vi "GAIN BASIC.vi"(0 "SR850 GPIB In":refnum<visa-resource-name>, 1 "Max. Hassasiyet":dbl=15.0, 2 "Auto Gain (False)":bool, 9 "Min. Hassasiyet":u16(ring) items=["100 nV", "200 nV", "500 nV", "1 uV", "2 uV", "5 uV", "10 uV", "20 uV", "50 uV", "100 uV", "200 uV", "500 uV", "1 mV"], 11 "error in":errorcluster) -> (4 "SR850 GPIB Out":refnum<visa-resource-name>, 15 "error out":errorcluster)   [LabVIEW 2014]
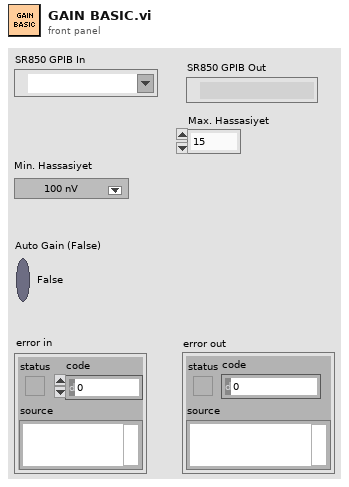
[diagram p1: front panel]
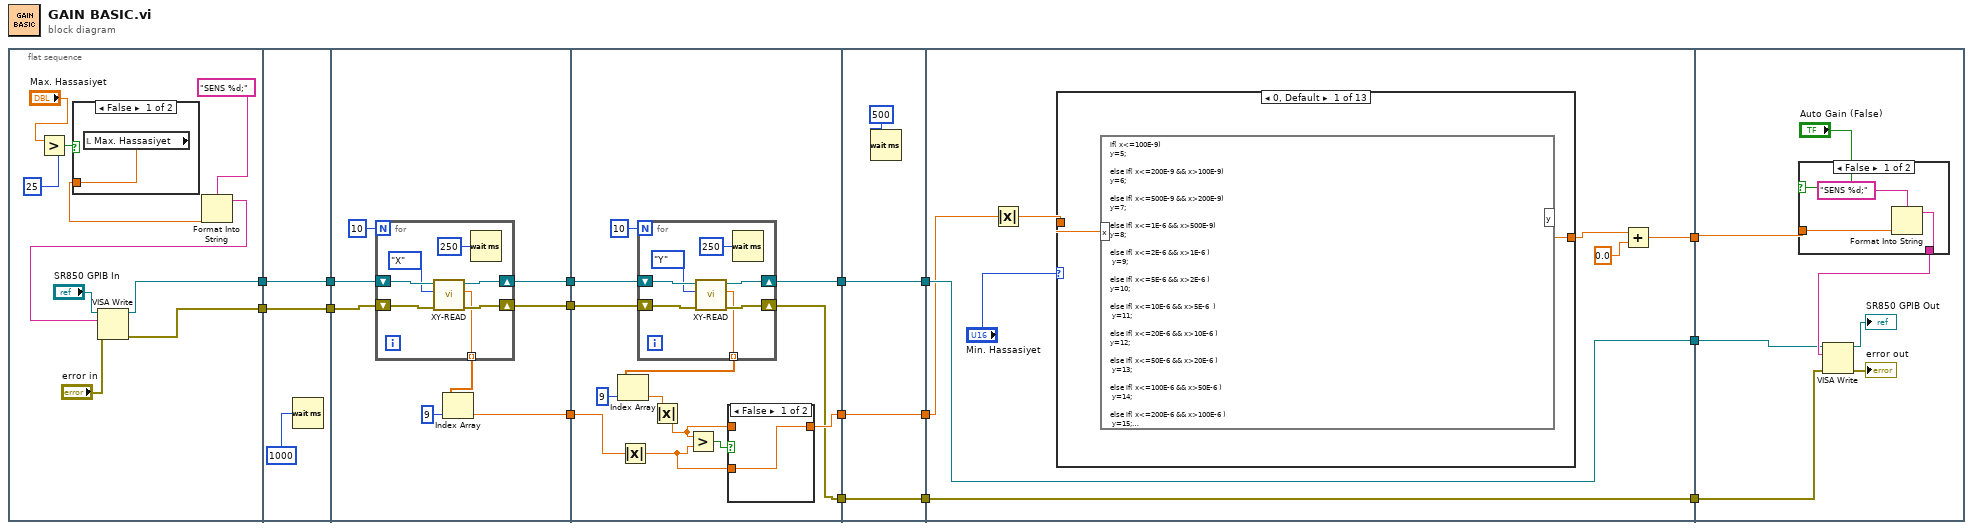
[diagram p0: block diagram]
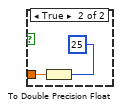
[diagram p2: hidden frame]
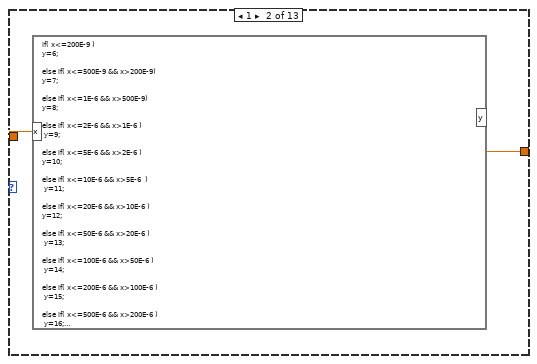
[diagram p4: hidden frame]
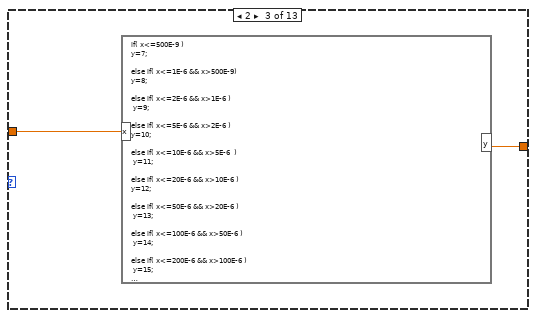
[diagram p5: hidden frame]
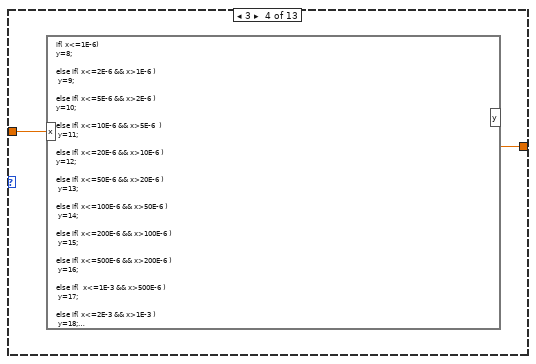
[diagram p6: hidden frame]
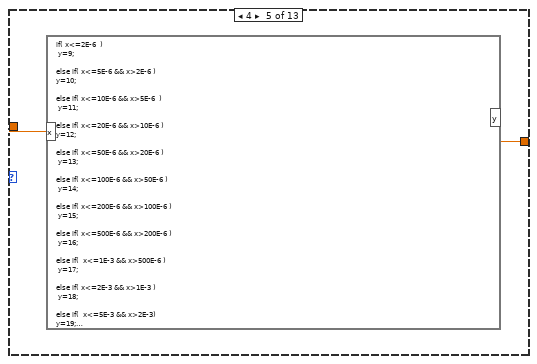
[diagram p7: hidden frame]
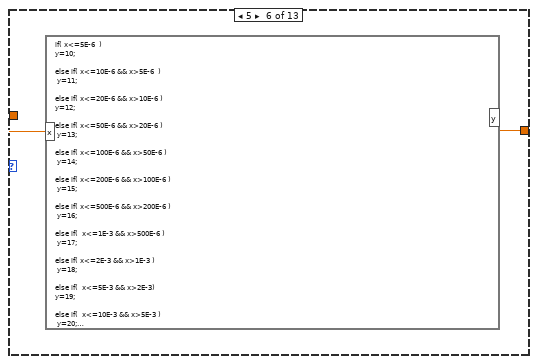
[diagram p8: hidden frame]
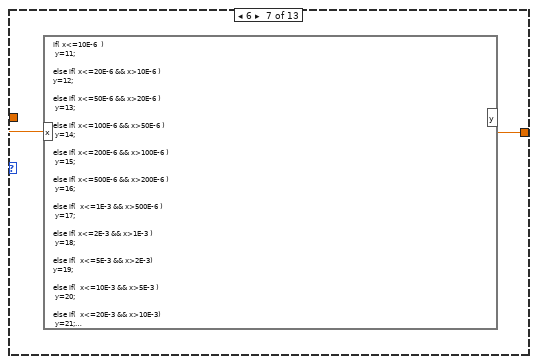
[diagram p9: hidden frame]
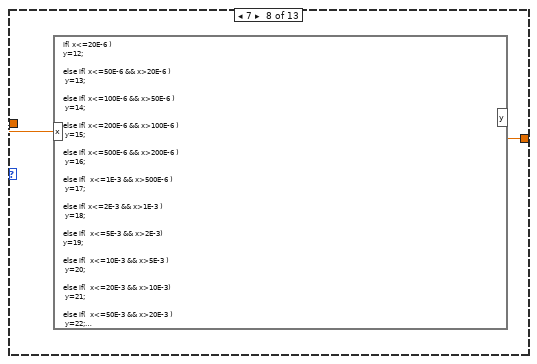
[diagram p10: hidden frame]
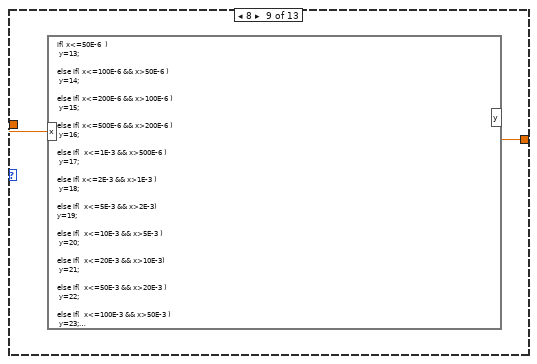
[diagram p11: hidden frame]
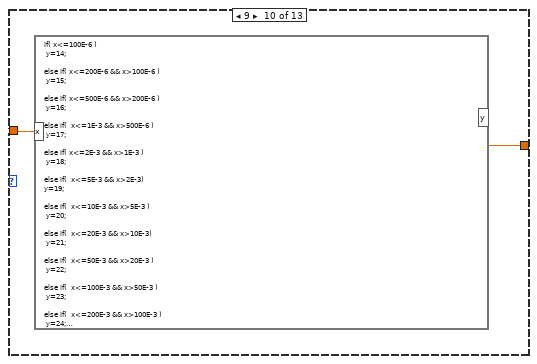
[diagram p12: hidden frame]
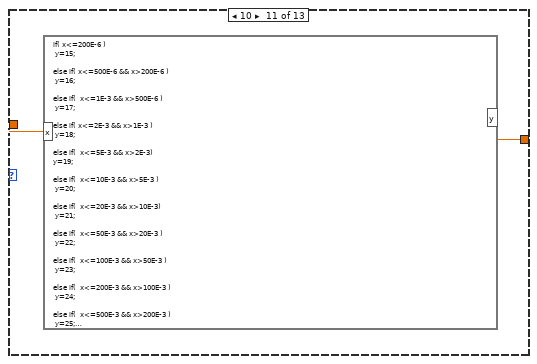
[diagram p13: hidden frame]
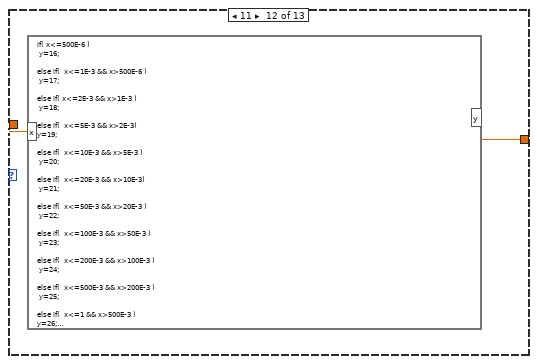
[diagram p14: hidden frame]
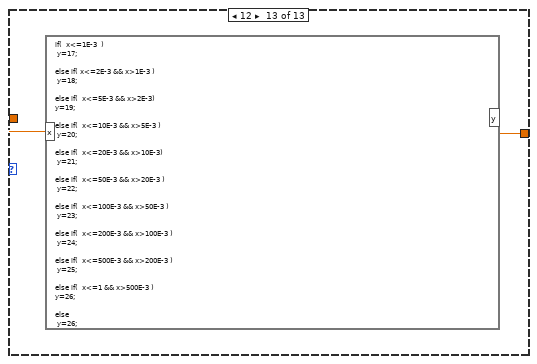
[diagram p15: hidden frame]
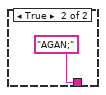
[diagram p16: hidden frame]
diagram:
  n1 = flat-sequence {
    tunnel: [w24] -> w13
    tunnel: [w21] -> w11
    tunnel: w13 -> [w32]
    tunnel: [w32] -> w12
    tunnel: w11 -> [w31]
    tunnel: [w31] -> w10
    tunnel: w12 -> [w40]
    tunnel: w10 -> [w39]
    tunnel: [w38] -> w6
    tunnel: [w34] -> w3
    tunnel: [w33] -> w1
    tunnel: w6 -> [w56]
    tunnel: [w57] -> w5
    tunnel: [w48] -> w4
    tunnel: w3 -> [w52]
    tunnel: [w51] -> w2
    tunnel: w1 -> [w55]
    tunnel: w5 -> [w73]
    tunnel: [w73] -> w9
    tunnel: w4 -> [w72]
    tunnel: [w72] -> w8
    tunnel: w2 -> [w71]
    tunnel: [w71] -> w7
    tunnel: [w80] -> w16
    tunnel: w9 -> [w80]
    tunnel: [w79] -> w15
    tunnel: w8 -> [w79]
    tunnel: w7 -> [w77]
    tunnel: [w74] -> w14
    tunnel: w16 -> [w109]
    tunnel: w15 -> [w108]
    tunnel: w14 -> [w110]
    frame #0 {
      n2 = Greater?(x="Max. Hassasiyet", y=25) -> (0:w18:bool)
      n3 = case shown="False" w18 {
        tunnel: [w27 w28] -> w17
        frame False {
          n4 = local read "Max. Hassasiyet"() -> (w27:dbl)
        }
        frame True {
          n5 = To Double Precision Float(number=25) -> (double precision float=w28:dbl)
        }
      }
      n6 = Format Into String(format string="SENS %d;", w17) -> (resulting string=w22:string)  [unwired: 2 in, 1 out]
      n7 = VISA Write(VISA resource name="SR850 GPIB In", write buffer=w22, error in (no error)="error in") -> (VISA resource name out=w24:refnum<visa-resource-name>, error out=w21:errorcluster)  [unwired: 1 out]
    }
    frame #1 {
      n8 = Wait (ms)(milliseconds to wait=u32 1000) -> ()  [unwired: 1 out]
    }
    frame #2 {
      n9 = for {
        N: 10 -> [_]
        shift-right: [w45] -> w38
        shift-left: w40 -> [w47]
        shift-right: [w44] -> w33
        shift-left: w39 -> [w46]
        tunnel: [w43] -> w36 mode=indexing
        n10 = call "XY-READ.vi"("Error IN"=w46, "X/Y ?"=enum16{"X", "Y"}."X", "SR850 GPIB IN"=w47) -> ("Error OUT"=w44:errorcluster, "SR850_Reading"=w43:dbl, "SR850 GPIB OUT"=w45:refnum<visa-resource-name>)  [unwired: 6 in]
        n11 = Wait (ms)(milliseconds to wait=u32 250) -> ()  [unwired: 1 out]
      }
      n12 = Index Array(array=w36, index=9) -> (element=w34:dbl)
    }
    frame #3 {
      n13 = Absolute Value(x=w52) -> (abs(x)=w49:dbl)
      n14 = for {
        N: 10 -> [_]
        shift-right: [w67] -> w57
        shift-left: w56 -> [w69]
        shift-right: [w66] -> w48
        shift-left: w55 -> [w68]
        tunnel: [w65] -> w59 mode=indexing
        n15 = call "XY-READ.vi"("Error IN"=w68, "X/Y ?"=enum16{"X", "Y"}."Y", "SR850 GPIB IN"=w69) -> ("Error OUT"=w66:errorcluster, "SR850_Reading"=w65:dbl, "SR850 GPIB OUT"=w67:refnum<visa-resource-name>)  [unwired: 6 in]
        n16 = Wait (ms)(milliseconds to wait=u32 250) -> ()  [unwired: 1 out]
      }
      n17 = Index Array(array=w59, index=9) -> (element=w53:dbl)
      n18 = Absolute Value(x=w53) -> (abs(x)=w50:dbl)
      n19 = Greater?(x=w50, y=w49) -> (0:w54:bool)
      n20 = case shown="False" w54 {
        tunnel: [w61 w62] -> w51
        tunnel: w50 -> [_ w62]
        tunnel: w49 -> [w61 _]
        frame False {
        }
        frame True {
        }
      }
    }
    frame #4 {
      n21 = Wait (ms)(milliseconds to wait=u32 500) -> ()  [unwired: 1 out]
    }
    frame #5 {
      n22 = Absolute Value(x=w77) -> (abs(x)=w78:dbl)
      n23 = case shown="0, Default" "Min. Hassasiyet" {
        tunnel: [w83 w85 w86 w89 w91 w93 w94 w96 w98 w100 w102 w104 w106] -> w76
        tunnel: w78 -> [w82 w84 w87 w88 w90 w92 w95 w97 w99 w101 w103 w105 w107]
        frame 0, Default {
          n24 = formula code="if( x<=100E-9) \ny=5;\n\nelse if( x<=200E-9 && x>100E-9) \ny=6;\n\nelse if( x<=500E-9 && x>200E-9) \ny=7;\n\nelse if( x<=1E-6 && x>500E-9) \ny=8;\n\nelse if( x<=2E-6 && x>1E-6 ) \n\ty=9;\n\nelse if( x<=5E-6 && x>2E-6 ) \ny=10;\n\nelse if( x<=10E-6 && x>5E-6  ) \n\ty=11;\n\nelse if( x<=20E-6 && x>10E-6 ) \ny=12;\n\nelse if( x<=50E-6 && x>20E-6 ) \n\ty=13;\n\nelse if( x<=100E-6 && x>50E-6 ) \n\ty=14;\n\nelse if( x<=200E-6 && x>100E-6 ) \n\ty=15;\n\nelse if( x<=500E-6 && x>200E-6 ) \n\ty=16;\n\nelse if(  x<=1E-3 && x>500E-6 ) \n\ty=17;\n\nelse if( x<=2E-3 && x>1E-3 ) \n\ty=18;\n\nelse if(  x<=5E-3 && x>2E-3) \ny=19;\n\nelse if(  x<=10E-3 && x>5E-3 ) \n\ty=20;\n\nelse if(  x<=20E-3 && x>10E-3) \n\ty=21;\n\nelse if(  x<=50E-3 && x>20E-3 ) \n\ty=22;\n\nelse if(  x<=100E-3 && x>50E-3 ) \n\ty=23;\n\nelse if(  x<=200E-3 && x>100E-3 ) \n\ty=24;\n\nelse if(  x<=500E-3 && x>200E-3 ) \n\ty=25;\n\nelse if(  x<=1 && x>500E-3 ) \ny=26;\n\nelse \n\ty=26;"("x"=w82) -> ("y"=w83:dbl)
        }
        frame 1 {
          n25 = formula code="if( x<=200E-9 ) \ny=6;\n\nelse if( x<=500E-9 && x>200E-9) \ny=7;\n\nelse if( x<=1E-6 && x>500E-9) \ny=8;\n\nelse if( x<=2E-6 && x>1E-6 ) \n\ty=9;\n\nelse if( x<=5E-6 && x>2E-6 ) \ny=10;\n\nelse if( x<=10E-6 && x>5E-6  ) \n\ty=11;\n\nelse if( x<=20E-6 && x>10E-6 ) \ny=12;\n\nelse if( x<=50E-6 && x>20E-6 ) \n\ty=13;\n\nelse if( x<=100E-6 && x>50E-6 ) \n\ty=14;\n\nelse if( x<=200E-6 && x>100E-6 ) \n\ty=15;\n\nelse if( x<=500E-6 && x>200E-6 ) \n\ty=16;\n\nelse if(  x<=1E-3 && x>500E-6 ) \n\ty=17;\n\nelse if( x<=2E-3 && x>1E-3 ) \n\ty=18;\n\nelse if(  x<=5E-3 && x>2E-3) \ny=19;\n\nelse if(  x<=10E-3 && x>5E-3 ) \n\ty=20;\n\nelse if(  x<=20E-3 && x>10E-3) \n\ty=21;\n\nelse if(  x<=50E-3 && x>20E-3 ) \n\ty=22;\n\nelse if(  x<=100E-3 && x>50E-3 ) \n\ty=23;\n\nelse if(  x<=200E-3 && x>100E-3 ) \n\ty=24;\n\nelse if(  x<=500E-3 && x>200E-3 ) \n\ty=25;\n\nelse if(  x<=1 && x>500E-3 ) \ny=26;\n\nelse \n\ty=26;"("x"=w84) -> ("y"=w85:dbl)
        }
        frame 2 {
          n26 = formula code="if( x<=500E-9 ) \ny=7;\n\nelse if( x<=1E-6 && x>500E-9) \ny=8;\n\nelse if( x<=2E-6 && x>1E-6 ) \n\ty=9;\n\nelse if( x<=5E-6 && x>2E-6 ) \ny=10;\n\nelse if( x<=10E-6 && x>5E-6  ) \n\ty=11;\n\nelse if( x<=20E-6 && x>10E-6 ) \ny=12;\n\nelse if( x<=50E-6 && x>20E-6 ) \n\ty=13;\n\nelse if( x<=100E-6 && x>50E-6 ) \n\ty=14;\n\nelse if( x<=200E-6 && x>100E-6 ) \n\ty=15;\n\nelse if( x<=500E-6 && x>200E-6 ) \n\ty=16;\n\nelse if(  x<=1E-3 && x>500E-6 ) \n\ty=17;\n\nelse if( x<=2E-3 && x>1E-3 ) \n\ty=18;\n\nelse if(  x<=5E-3 && x>2E-3) \ny=19;\n\nelse if(  x<=10E-3 && x>5E-3 ) \n\ty=20;\n\nelse if(  x<=20E-3 && x>10E-3) \n\ty=21;\n\nelse if(  x<=50E-3 && x>20E-3 ) \n\ty=22;\n\nelse if(  x<=100E-3 && x>50E-3 ) \n\ty=23;\n\nelse if(  x<=200E-3 && x>100E-3 ) \n\ty=24;\n\nelse if(  x<=500E-3 && x>200E-3 ) \n\ty=25;\n\nelse if(  x<=1 && x>500E-3 ) \ny=26;\n\nelse \n\ty=26;"("x"=w87) -> ("y"=w86:dbl)
        }
        frame 3 {
          n27 = formula code="if( x<=1E-6) \ny=8;\n\nelse if( x<=2E-6 && x>1E-6 ) \n\ty=9;\n\nelse if( x<=5E-6 && x>2E-6 ) \ny=10;\n\nelse if( x<=10E-6 && x>5E-6  ) \n\ty=11;\n\nelse if( x<=20E-6 && x>10E-6 ) \ny=12;\n\nelse if( x<=50E-6 && x>20E-6 ) \n\ty=13;\n\nelse if( x<=100E-6 && x>50E-6 ) \n\ty=14;\n\nelse if( x<=200E-6 && x>100E-6 ) \n\ty=15;\n\nelse if( x<=500E-6 && x>200E-6 ) \n\ty=16;\n\nelse if(  x<=1E-3 && x>500E-6 ) \n\ty=17;\n\nelse if( x<=2E-3 && x>1E-3 ) \n\ty=18;\n\nelse if(  x<=5E-3 && x>2E-3) \ny=19;\n\nelse if(  x<=10E-3 && x>5E-3 ) \n\ty=20;\n\nelse if(  x<=20E-3 && x>10E-3) \n\ty=21;\n\nelse if(  x<=50E-3 && x>20E-3 ) \n\ty=22;\n\nelse if(  x<=100E-3 && x>50E-3 ) \n\ty=23;\n\nelse if(  x<=200E-3 && x>100E-3 ) \n\ty=24;\n\nelse if(  x<=500E-3 && x>200E-3 ) \n\ty=25;\n\nelse if(  x<=1 && x>500E-3 ) \ny=26;\n\nelse \n\ty=26;"("x"=w88) -> ("y"=w89:dbl)
        }
        frame 4 {
          n28 = formula code="if( x<=2E-6  ) \n\ty=9;\n\nelse if( x<=5E-6 && x>2E-6 ) \ny=10;\n\nelse if( x<=10E-6 && x>5E-6  ) \n\ty=11;\n\nelse if( x<=20E-6 && x>10E-6 ) \ny=12;\n\nelse if( x<=50E-6 && x>20E-6 ) \n\ty=13;\n\nelse if( x<=100E-6 && x>50E-6 ) \n\ty=14;\n\nelse if( x<=200E-6 && x>100E-6 ) \n\ty=15;\n\nelse if( x<=500E-6 && x>200E-6 ) \n\ty=16;\n\nelse if(  x<=1E-3 && x>500E-6 ) \n\ty=17;\n\nelse if( x<=2E-3 && x>1E-3 ) \n\ty=18;\n\nelse if(  x<=5E-3 && x>2E-3) \ny=19;\n\nelse if(  x<=10E-3 && x>5E-3 ) \n\ty=20;\n\nelse if(  x<=20E-3 && x>10E-3) \n\ty=21;\n\nelse if(  x<=50E-3 && x>20E-3 ) \n\ty=22;\n\nelse if(  x<=100E-3 && x>50E-3 ) \n\ty=23;\n\nelse if(  x<=200E-3 && x>100E-3 ) \n\ty=24;\n\nelse if(  x<=500E-3 && x>200E-3 ) \n\ty=25;\n\nelse if(  x<=1 && x>500E-3 ) \ny=26;\n\nelse \n\ty=26;"("x"=w90) -> ("y"=w91:dbl)
        }
        frame 5 {
          n29 = formula code="if( x<=5E-6  ) \ny=10;\n\nelse if( x<=10E-6 && x>5E-6  ) \n\ty=11;\n\nelse if( x<=20E-6 && x>10E-6 ) \ny=12;\n\nelse if( x<=50E-6 && x>20E-6 ) \n\ty=13;\n\nelse if( x<=100E-6 && x>50E-6 ) \n\ty=14;\n\nelse if( x<=200E-6 && x>100E-6 ) \n\ty=15;\n\nelse if( x<=500E-6 && x>200E-6 ) \n\ty=16;\n\nelse if(  x<=1E-3 && x>500E-6 ) \n\ty=17;\n\nelse if( x<=2E-3 && x>1E-3 ) \n\ty=18;\n\nelse if(  x<=5E-3 && x>2E-3) \ny=19;\n\nelse if(  x<=10E-3 && x>5E-3 ) \n\ty=20;\n\nelse if(  x<=20E-3 && x>10E-3) \n\ty=21;\n\nelse if(  x<=50E-3 && x>20E-3 ) \n\ty=22;\n\nelse if(  x<=100E-3 && x>50E-3 ) \n\ty=23;\n\nelse if(  x<=200E-3 && x>100E-3 ) \n\ty=24;\n\nelse if(  x<=500E-3 && x>200E-3 ) \n\ty=25;\n\nelse if(  x<=1 && x>500E-3 ) \ny=26;\n\nelse \n\ty=26;"("x"=w92) -> ("y"=w93:dbl)
        }
        frame 6 {
          n30 = formula code="if( x<=10E-6  ) \n\ty=11;\n\nelse if( x<=20E-6 && x>10E-6 ) \ny=12;\n\nelse if( x<=50E-6 && x>20E-6 ) \n\ty=13;\n\nelse if( x<=100E-6 && x>50E-6 ) \n\ty=14;\n\nelse if( x<=200E-6 && x>100E-6 ) \n\ty=15;\n\nelse if( x<=500E-6 && x>200E-6 ) \n\ty=16;\n\nelse if(  x<=1E-3 && x>500E-6 ) \n\ty=17;\n\nelse if( x<=2E-3 && x>1E-3 ) \n\ty=18;\n\nelse if(  x<=5E-3 && x>2E-3) \ny=19;\n\nelse if(  x<=10E-3 && x>5E-3 ) \n\ty=20;\n\nelse if(  x<=20E-3 && x>10E-3) \n\ty=21;\n\nelse if(  x<=50E-3 && x>20E-3 ) \n\ty=22;\n\nelse if(  x<=100E-3 && x>50E-3 ) \n\ty=23;\n\nelse if(  x<=200E-3 && x>100E-3 ) \n\ty=24;\n\nelse if(  x<=500E-3 && x>200E-3 ) \n\ty=25;\n\nelse if(  x<=1 && x>500E-3 ) \ny=26;\n\nelse \n\ty=26;"("x"=w95) -> ("y"=w94:dbl)
        }
        frame 7 {
          n31 = formula code="if( x<=20E-6 ) \ny=12;\n\nelse if( x<=50E-6 && x>20E-6 ) \n\ty=13;\n\nelse if( x<=100E-6 && x>50E-6 ) \n\ty=14;\n\nelse if( x<=200E-6 && x>100E-6 ) \n\ty=15;\n\nelse if( x<=500E-6 && x>200E-6 ) \n\ty=16;\n\nelse if(  x<=1E-3 && x>500E-6 ) \n\ty=17;\n\nelse if( x<=2E-3 && x>1E-3 ) \n\ty=18;\n\nelse if(  x<=5E-3 && x>2E-3) \ny=19;\n\nelse if(  x<=10E-3 && x>5E-3 ) \n\ty=20;\n\nelse if(  x<=20E-3 && x>10E-3) \n\ty=21;\n\nelse if(  x<=50E-3 && x>20E-3 ) \n\ty=22;\n\nelse if(  x<=100E-3 && x>50E-3 ) \n\ty=23;\n\nelse if(  x<=200E-3 && x>100E-3 ) \n\ty=24;\n\nelse if(  x<=500E-3 && x>200E-3 ) \n\ty=25;\n\nelse if(  x<=1 && x>500E-3 ) \ny=26;\n\nelse \n\ty=26;"("x"=w97) -> ("y"=w96:dbl)
        }
        frame 8 {
          n32 = formula code="if( x<=50E-6  ) \n\ty=13;\n\nelse if( x<=100E-6 && x>50E-6 ) \n\ty=14;\n\nelse if( x<=200E-6 && x>100E-6 ) \n\ty=15;\n\nelse if( x<=500E-6 && x>200E-6 ) \n\ty=16;\n\nelse if(  x<=1E-3 && x>500E-6 ) \n\ty=17;\n\nelse if( x<=2E-3 && x>1E-3 ) \n\ty=18;\n\nelse if(  x<=5E-3 && x>2E-3) \ny=19;\n\nelse if(  x<=10E-3 && x>5E-3 ) \n\ty=20;\n\nelse if(  x<=20E-3 && x>10E-3) \n\ty=21;\n\nelse if(  x<=50E-3 && x>20E-3 ) \n\ty=22;\n\nelse if(  x<=100E-3 && x>50E-3 ) \n\ty=23;\n\nelse if(  x<=200E-3 && x>100E-3 ) \n\ty=24;\n\nelse if(  x<=500E-3 && x>200E-3 ) \n\ty=25;\n\nelse if(  x<=1 && x>500E-3 ) \ny=26;\n\nelse \n\ty=26;"("x"=w99) -> ("y"=w98:dbl)
        }
        frame 9 {
          n33 = formula code="if( x<=100E-6 ) \n\ty=14;\n\nelse if( x<=200E-6 && x>100E-6 ) \n\ty=15;\n\nelse if( x<=500E-6 && x>200E-6 ) \n\ty=16;\n\nelse if(  x<=1E-3 && x>500E-6 ) \n\ty=17;\n\nelse if( x<=2E-3 && x>1E-3 ) \n\ty=18;\n\nelse if(  x<=5E-3 && x>2E-3) \ny=19;\n\nelse if(  x<=10E-3 && x>5E-3 ) \n\ty=20;\n\nelse if(  x<=20E-3 && x>10E-3) \n\ty=21;\n\nelse if(  x<=50E-3 && x>20E-3 ) \n\ty=22;\n\nelse if(  x<=100E-3 && x>50E-3 ) \n\ty=23;\n\nelse if(  x<=200E-3 && x>100E-3 ) \n\ty=24;\n\nelse if(  x<=500E-3 && x>200E-3 ) \n\ty=25;\n\nelse if(  x<=1 && x>500E-3 ) \ny=26;\n\nelse \n\ty=26;"("x"=w101) -> ("y"=w100:dbl)
        }
        frame 10 {
          n34 = formula code="if( x<=200E-6 ) \n\ty=15;\n\nelse if( x<=500E-6 && x>200E-6 ) \n\ty=16;\n\nelse if(  x<=1E-3 && x>500E-6 ) \n\ty=17;\n\nelse if( x<=2E-3 && x>1E-3 ) \n\ty=18;\n\nelse if(  x<=5E-3 && x>2E-3) \ny=19;\n\nelse if(  x<=10E-3 && x>5E-3 ) \n\ty=20;\n\nelse if(  x<=20E-3 && x>10E-3) \n\ty=21;\n\nelse if(  x<=50E-3 && x>20E-3 ) \n\ty=22;\n\nelse if(  x<=100E-3 && x>50E-3 ) \n\ty=23;\n\nelse if(  x<=200E-3 && x>100E-3 ) \n\ty=24;\n\nelse if(  x<=500E-3 && x>200E-3 ) \n\ty=25;\n\nelse if(  x<=1 && x>500E-3 ) \ny=26;\n\nelse \n\ty=26;"("x"=w103) -> ("y"=w102:dbl)
        }
        frame 11 {
          n35 = formula code="if( x<=500E-6 ) \n\ty=16;\n\nelse if(  x<=1E-3 && x>500E-6 ) \n\ty=17;\n\nelse if( x<=2E-3 && x>1E-3 ) \n\ty=18;\n\nelse if(  x<=5E-3 && x>2E-3) \ny=19;\n\nelse if(  x<=10E-3 && x>5E-3 ) \n\ty=20;\n\nelse if(  x<=20E-3 && x>10E-3) \n\ty=21;\n\nelse if(  x<=50E-3 && x>20E-3 ) \n\ty=22;\n\nelse if(  x<=100E-3 && x>50E-3 ) \n\ty=23;\n\nelse if(  x<=200E-3 && x>100E-3 ) \n\ty=24;\n\nelse if(  x<=500E-3 && x>200E-3 ) \n\ty=25;\n\nelse if(  x<=1 && x>500E-3 ) \ny=26;\n\nelse \n\ty=26;"("x"=w105) -> ("y"=w104:dbl)
        }
        frame 12 {
          n36 = formula code="if(  x<=1E-3  ) \n\ty=17;\n\nelse if( x<=2E-3 && x>1E-3 ) \n\ty=18;\n\nelse if(  x<=5E-3 && x>2E-3) \ny=19;\n\nelse if(  x<=10E-3 && x>5E-3 ) \n\ty=20;\n\nelse if(  x<=20E-3 && x>10E-3) \n\ty=21;\n\nelse if(  x<=50E-3 && x>20E-3 ) \n\ty=22;\n\nelse if(  x<=100E-3 && x>50E-3 ) \n\ty=23;\n\nelse if(  x<=200E-3 && x>100E-3 ) \n\ty=24;\n\nelse if(  x<=500E-3 && x>200E-3 ) \n\ty=25;\n\nelse if(  x<=1 && x>500E-3 ) \ny=26;\n\nelse \n\ty=26;"("x"=w107) -> ("y"=w106:dbl)
        }
      }
      n37 = Add(x=w76, y=0.0) -> (x+y=w74:dbl)
    }
    frame #6 {
      n38 = case shown="False" "Auto Gain (False)" {
        tunnel: [w116 "AGAN;" ("true string")] -> w111
        tunnel: w110 -> [w115 _]
        frame False {
          n39 = Format Into String(format string="SENS %d;", w115) -> (resulting string=w116:string)  [unwired: 2 in, 1 out]
        }
        frame True {
        }
      }
      n40 = VISA Write(VISA resource name=w109, write buffer=w111, error in (no error)=w108) -> (VISA resource name out=→"SR850 GPIB Out":refnum<visa-resource-name>, error out=→"error out":errorcluster)  [unwired: 1 out]
    }
  }
